vi "Run.vi"(8 "error in (no error)":errorcluster, 11 "Channel GUI in":refnum<class "Channel.lvclass">) -> (0 "error out":errorcluster, 3 "Channel GUI out":refnum<class "Channel.lvclass">)   [LabVIEW 2018, in "Channel.lvclass"]
uses:
  Channel.lvclass
  Channel.lvclass/Channel.ctl
  State Machine/State Machine.lvclass
  Camera/Camera.lvclass
  Request/Request.lvclass
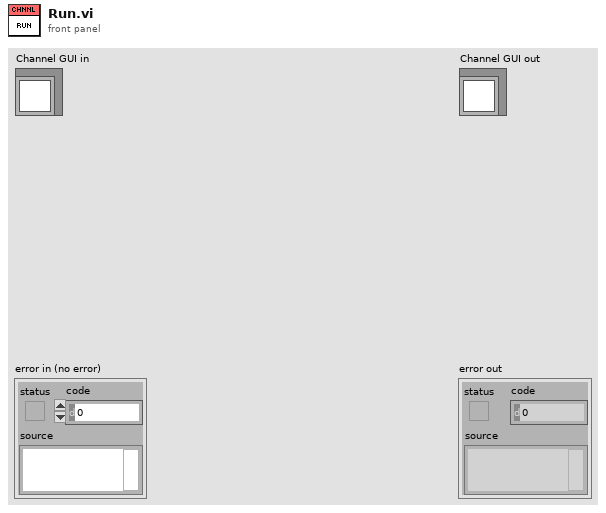
[diagram p1: front panel]
types:
  T1 = cluster{"PREAMP":u16, "READOUT_RATE":u16, "VERTICAL_SHIFT_SPEED":u16, "READ_MODE":u16, "VERTICAL_CLOCK_VOLTAGE":u16, "ACQUISITION_MODE":u16, "AD_CHANNEL":u16, "SHUTTER_TTL":u16, "SHUTTER_OPENING_TIME":u16, "SHUTTER_CLOSING_TIME":u16, "SHUTTER_MODE":u16, "TRIGGER_MODE":u16, "VBIN":u16, "INITIAL_LINE":u16, "INITIAL_COLUMN":u16, "FINAL_LINE":u16, "FINAL_COLUMN":u16, "HBIN":u16, "HIGH_CAPACITY":bool, "COOLER":u16, "TEMP":u16}
  T2 = cluster{"device":string, "action":string, "parameter":string}
  T3 = cluster{"EXPTIME":dbl, "#FRAMES":u32, "#CYCLES":u32, "suffix":string}
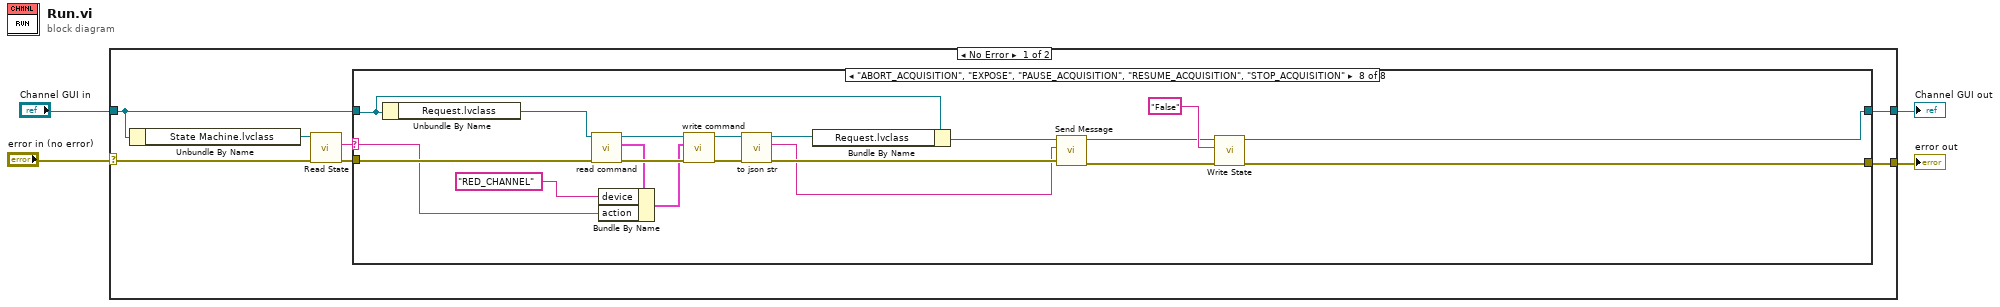
[diagram p0: block diagram]
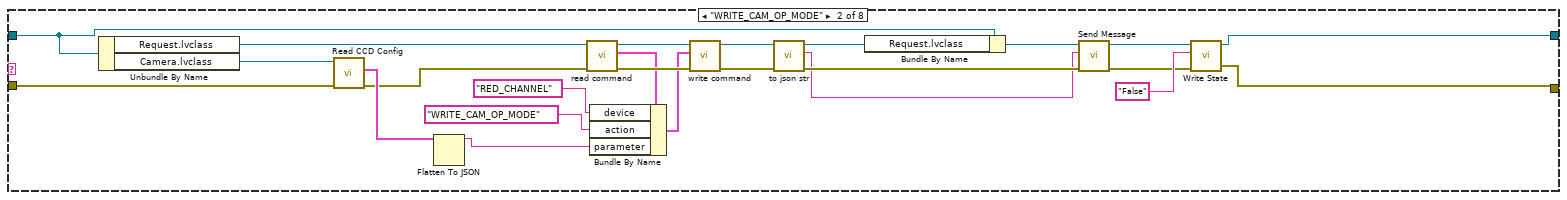
[diagram p3: hidden frame]
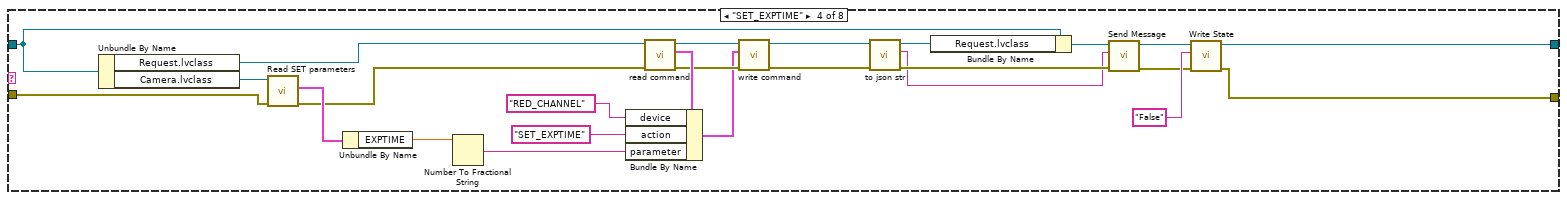
[diagram p5: hidden frame]
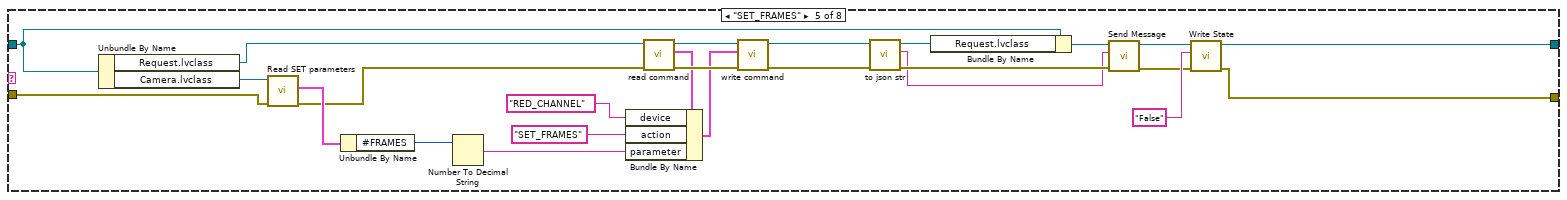
[diagram p6: hidden frame]
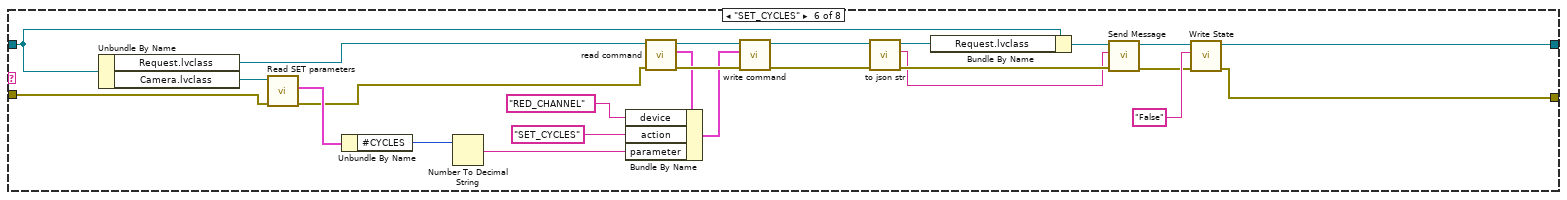
[diagram p7: hidden frame]
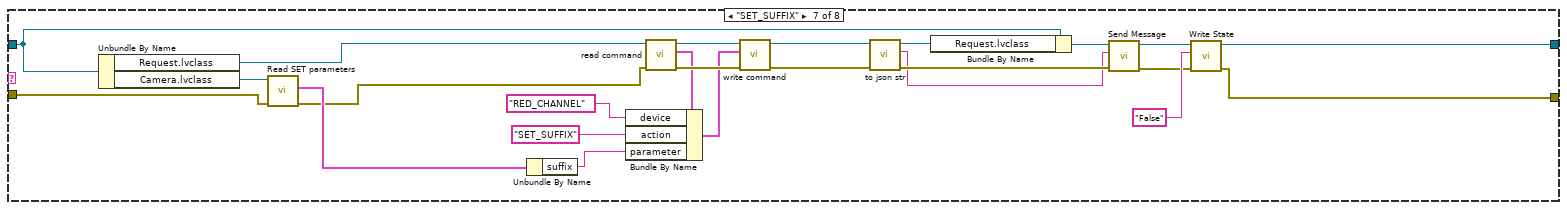
[diagram p8: hidden frame]
diagram:
  n1 = case shown="No Error" "error in (no error)" {
    selector: "error in (no error)" -> [w9 w160]
    tunnel: [w11 w160] -> w2
    tunnel: "Channel GUI in" -> [w7 w159]
    tunnel: [w6 w159] -> w1
    frame No Error {
      n2 = Unbundle By Name(w7) -> ("State Machine.lvclass"=w10:refnum<class "State Machine.lvclass">)
      n3 = call-dynamic "Read State.vi"("error in (no error)"=w9, "State Machine in"=w10) -> ("error out"=w8:errorcluster, "State"=w5:string)  [unwired: 7 in, 1 out]
      n4 = case shown="\"ABORT_ACQUISITION\", \"EXPOSE\", \"PAUSE_ACQUISITION\", \"RESUME_ACQUISITION\", \"STOP_ACQUISITION\"" w5 {
        selector: w5 -> [_ _ _ _ _ _ _ w139]
        tunnel: w8 -> [w13 w36 w38 w63 w88 w113 w137 w150]
        tunnel: [w13 w32 w38 w58 w83 w108 w132 w157] -> w11
        tunnel: w7 -> [w12 w21 w39 w55 w80 w105 w129 w145]
        tunnel: [w12 w33 w39 w59 w84 w109 w133 w154] -> w6
        frame "False", Default {
        }
        frame "WRITE_CAM_OP_MODE" {
          n5 = Unbundle By Name(w21) -> ("Request.lvclass"=w27:refnum<class "Request.lvclass">, "Camera.lvclass"=w37:refnum<class "Camera.lvclass">)
          n6 = call-dynamic "Read CCD Config.vi"("error in (no error)"=w36, "Camera in"=w37) -> ("error out"=w22:errorcluster, "CCD Config"=w35:T1)  [unwired: 7 in, 1 out]
          n7 = Flatten To JSON(anything=w35) -> (JSON string=w14:string)  [unwired: 2 in, 1 out]
          n8 = call "read command.vi"("error in (no error)"=w22, "Request in"=w27) -> ("error out"=w28:errorcluster, "command"=w26:T2, "Request out"=w29:refnum<class "Request.lvclass">)  [unwired: 7 in]
          n9 = Bundle By Name(cluster=w26, "device"="RED_CHANNEL", "action"="WRITE_CAM_OP_MODE", "parameter"=w14) -> (w25:T2)
          n10 = call "write command.vi"("error in (no error)"=w28, "command"=w25, "Request in"=w29) -> ("error out"=w18:errorcluster, "Request out"=w19:refnum<class "Request.lvclass">)  [unwired: 7 in]
          n11 = call "to json str.vi"("error in (no error)"=w18, "Request in"=w19) -> ("error out"=w17:errorcluster, "request str"=w15:string, "Request out"=w16:refnum<class "Request.lvclass">)  [unwired: 7 in]
          n12 = Bundle By Name(cluster=w21, "Request.lvclass"=w16) -> (w20:refnum<class "Channel.lvclass">)
          n13 = call "Send Message.vi"("error in (no error)"=w17, "Message"=w15, "Channel GUI in"=w20) -> ("error out"=w31:errorcluster, "Channel GUI out"=w30:refnum<class "Channel.lvclass">)  [unwired: 7 in]
          n14 = call "Write State.vi"("error in (no error)"=w31, "State"="False" ("New_State"), "Channel GEI in"=w30) -> ("error out"=w32:errorcluster, "Channel GEI out"=w33:refnum<class "Channel.lvclass">)  [unwired: 7 in]
        }
        frame "--------------------------" {
        }
        frame "SET_EXPTIME" {
          n15 = Unbundle By Name(w55) -> ("Request.lvclass"=w40:refnum<class "Request.lvclass">, "Camera.lvclass"=w64:refnum<class "Camera.lvclass">)
          n16 = call-dynamic "Read SET parameters.vi"("error in (no error)"=w63, "Camera in"=w64) -> ("error out"=w41:errorcluster, "SET parameters"=w62:T3)  [unwired: 7 in, 1 out]
          n17 = Unbundle By Name(w62) -> ("EXPTIME"=w61:dbl)
          n18 = Number To Fractional String(number=w61) -> (F-format string=w48:string)  [unwired: 3 in]
          n19 = call "read command.vi"("error in (no error)"=w41, "Request in"=w40) -> ("error out"=w45:errorcluster, "command"=w47:T2, "Request out"=w46:refnum<class "Request.lvclass">)  [unwired: 7 in]
          n20 = Bundle By Name(cluster=w47, "device"="RED_CHANNEL", "action"="SET_EXPTIME", "parameter"=w48) -> (w44:T2)
          n21 = call "write command.vi"("error in (no error)"=w45, "command"=w44, "Request in"=w46) -> ("error out"=w43:errorcluster, "Request out"=w42:refnum<class "Request.lvclass">)  [unwired: 7 in]
          n22 = call "to json str.vi"("error in (no error)"=w43, "Request in"=w42) -> ("error out"=w52:errorcluster, "request str"=w51:string, "Request out"=w53:refnum<class "Request.lvclass">)  [unwired: 7 in]
          n23 = Bundle By Name(cluster=w55, "Request.lvclass"=w53) -> (w54:refnum<class "Channel.lvclass">)
          n24 = call "Send Message.vi"("error in (no error)"=w52, "Message"=w51, "Channel GUI in"=w54) -> ("error out"=w57:errorcluster, "Channel GUI out"=w56:refnum<class "Channel.lvclass">)  [unwired: 7 in]
          n25 = call "Write State.vi"("error in (no error)"=w57, "State"="False" ("New_State"), "Channel GEI in"=w56) -> ("error out"=w58:errorcluster, "Channel GEI out"=w59:refnum<class "Channel.lvclass">)  [unwired: 7 in]
        }
        frame "SET_FRAMES" {
          n26 = Unbundle By Name(w80) -> ("Request.lvclass"=w65:refnum<class "Request.lvclass">, "Camera.lvclass"=w89:refnum<class "Camera.lvclass">)
          n27 = call-dynamic "Read SET parameters.vi"("error in (no error)"=w88, "Camera in"=w89) -> ("error out"=w66:errorcluster, "SET parameters"=w87:T3)  [unwired: 7 in, 1 out]
          n28 = Unbundle By Name(w87) -> ("#FRAMES"=w86:u32)
          n29 = Number To Decimal String(number=w86) -> (decimal integer string=w73:string)  [unwired: 1 in]
          n30 = call "read command.vi"("error in (no error)"=w66, "Request in"=w65) -> ("error out"=w71:errorcluster, "command"=w70:T2, "Request out"=w72:refnum<class "Request.lvclass">)  [unwired: 7 in]
          n31 = Bundle By Name(cluster=w70, "device"="RED_CHANNEL", "action"="SET_FRAMES", "parameter"=w73) -> (w69:T2)
          n32 = call "write command.vi"("error in (no error)"=w71, "command"=w69, "Request in"=w72) -> ("error out"=w67:errorcluster, "Request out"=w68:refnum<class "Request.lvclass">)  [unwired: 7 in]
          n33 = call "to json str.vi"("error in (no error)"=w67, "Request in"=w68) -> ("error out"=w77:errorcluster, "request str"=w76:string, "Request out"=w78:refnum<class "Request.lvclass">)  [unwired: 7 in]
          n34 = Bundle By Name(cluster=w80, "Request.lvclass"=w78) -> (w79:refnum<class "Channel.lvclass">)
          n35 = call "Send Message.vi"("error in (no error)"=w77, "Message"=w76, "Channel GUI in"=w79) -> ("error out"=w82:errorcluster, "Channel GUI out"=w81:refnum<class "Channel.lvclass">)  [unwired: 7 in]
          n36 = call "Write State.vi"("error in (no error)"=w82, "State"="False" ("New_State"), "Channel GEI in"=w81) -> ("error out"=w83:errorcluster, "Channel GEI out"=w84:refnum<class "Channel.lvclass">)  [unwired: 7 in]
        }
        frame "SET_CYCLES" {
          n37 = Unbundle By Name(w105) -> ("Request.lvclass"=w94:refnum<class "Request.lvclass">, "Camera.lvclass"=w114:refnum<class "Camera.lvclass">)
          n38 = call-dynamic "Read SET parameters.vi"("error in (no error)"=w113, "Camera in"=w114) -> ("error out"=w93:errorcluster, "SET parameters"=w112:T3)  [unwired: 7 in, 1 out]
          n39 = Unbundle By Name(w112) -> ("#CYCLES"=w111:u32)
          n40 = Number To Decimal String(number=w111) -> (decimal integer string=w98:string)  [unwired: 1 in]
          n41 = call "read command.vi"("error in (no error)"=w93, "Request in"=w94) -> ("error out"=w96:errorcluster, "command"=w95:T2, "Request out"=w97:refnum<class "Request.lvclass">)  [unwired: 7 in]
          n42 = Bundle By Name(cluster=w95, "device"="RED_CHANNEL", "action"="SET_CYCLES", "parameter"=w98) -> (w90:T2)
          n43 = call "write command.vi"("error in (no error)"=w96, "command"=w90, "Request in"=w97) -> ("error out"=w92:errorcluster, "Request out"=w91:refnum<class "Request.lvclass">)  [unwired: 7 in]
          n44 = call "to json str.vi"("error in (no error)"=w92, "Request in"=w91) -> ("error out"=w102:errorcluster, "request str"=w101:string, "Request out"=w103:refnum<class "Request.lvclass">)  [unwired: 7 in]
          n45 = Bundle By Name(cluster=w105, "Request.lvclass"=w103) -> (w104:refnum<class "Channel.lvclass">)
          n46 = call "Send Message.vi"("error in (no error)"=w102, "Message"=w101, "Channel GUI in"=w104) -> ("error out"=w107:errorcluster, "Channel GUI out"=w106:refnum<class "Channel.lvclass">)  [unwired: 7 in]
          n47 = call "Write State.vi"("error in (no error)"=w107, "State"="False" ("New_State"), "Channel GEI in"=w106) -> ("error out"=w108:errorcluster, "Channel GEI out"=w109:refnum<class "Channel.lvclass">)  [unwired: 7 in]
        }
        frame "SET_SUFFIX" {
          n48 = Unbundle By Name(w129) -> ("Request.lvclass"=w119:refnum<class "Request.lvclass">, "Camera.lvclass"=w138:refnum<class "Camera.lvclass">)
          n49 = call-dynamic "Read SET parameters.vi"("error in (no error)"=w137, "Camera in"=w138) -> ("error out"=w118:errorcluster, "SET parameters"=w136:T3)  [unwired: 7 in, 1 out]
          n50 = Unbundle By Name(w136) -> ("suffix"=w135:string)
          n51 = call "read command.vi"("error in (no error)"=w118, "Request in"=w119) -> ("error out"=w121:errorcluster, "command"=w120:T2, "Request out"=w122:refnum<class "Request.lvclass">)  [unwired: 7 in]
          n52 = Bundle By Name(cluster=w120, "device"="RED_CHANNEL", "action"="SET_SUFFIX", "parameter"=w135) -> (w115:T2)
          n53 = call "write command.vi"("error in (no error)"=w121, "command"=w115, "Request in"=w122) -> ("error out"=w117:errorcluster, "Request out"=w116:refnum<class "Request.lvclass">)  [unwired: 7 in]
          n54 = call "to json str.vi"("error in (no error)"=w117, "Request in"=w116) -> ("error out"=w126:errorcluster, "request str"=w125:string, "Request out"=w127:refnum<class "Request.lvclass">)  [unwired: 7 in]
          n55 = Bundle By Name(cluster=w129, "Request.lvclass"=w127) -> (w128:refnum<class "Channel.lvclass">)
          n56 = call "Send Message.vi"("error in (no error)"=w126, "Message"=w125, "Channel GUI in"=w128) -> ("error out"=w131:errorcluster, "Channel GUI out"=w130:refnum<class "Channel.lvclass">)  [unwired: 7 in]
          n57 = call "Write State.vi"("error in (no error)"=w131, "State"="False" ("New_State"), "Channel GEI in"=w130) -> ("error out"=w132:errorcluster, "Channel GEI out"=w133:refnum<class "Channel.lvclass">)  [unwired: 7 in]
        }
        frame "ABORT_ACQUISITION", "EXPOSE", "PAUSE_ACQUISITION", "RESUME_ACQUISITION", "STOP_ACQUISITION" {
          n58 = Unbundle By Name(w145) -> ("Request.lvclass"=w148:refnum<class "Request.lvclass">)
          n59 = call "read command.vi"("error in (no error)"=w150, "Request in"=w148) -> ("error out"=w152:errorcluster, "command"=w141:T2, "Request out"=w147:refnum<class "Request.lvclass">)  [unwired: 7 in]
          n60 = Bundle By Name(cluster=w141, "device"="RED_CHANNEL", "action"=w139) -> (w140:T2)
          n61 = call "write command.vi"("error in (no error)"=w152, "command"=w140, "Request in"=w147) -> ("error out"=w151:errorcluster, "Request out"=w146:refnum<class "Request.lvclass">)  [unwired: 7 in]
          n62 = call "to json str.vi"("error in (no error)"=w151, "Request in"=w146) -> ("error out"=w149:errorcluster, "request str"=w142:string, "Request out"=w143:refnum<class "Request.lvclass">)  [unwired: 7 in]
          n63 = Bundle By Name(cluster=w145, "Request.lvclass"=w143) -> (w144:refnum<class "Channel.lvclass">)
          n64 = call "Send Message.vi"("error in (no error)"=w149, "Message"=w142, "Channel GUI in"=w144) -> ("error out"=w156:errorcluster, "Channel GUI out"=w155:refnum<class "Channel.lvclass">)  [unwired: 7 in]
          n65 = call "Write State.vi"("error in (no error)"=w156, "State"="False", "Channel GEI in"=w155) -> ("error out"=w157:errorcluster, "Channel GEI out"=w154:refnum<class "Channel.lvclass">)  [unwired: 7 in]
        }
      }
    }
    frame Error {
    }
  }
  "error out" <- w2
  "Channel GUI out" <- w1
